vi "TPNT_ModifyDeviceTP.vi"(8 "error in (no error)":errorcluster, 9 "name":string, 10 "arguments":string, 11 "Object Refnum In":T1) -> (0 "error out":errorcluster, 3 "Data Refnum out":T1)   [LabVIEW 2016]
uses:
  TPNT_Refnum.ctl
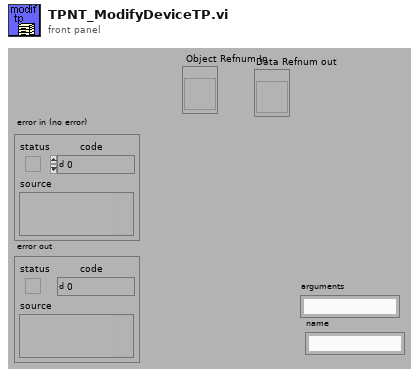
[diagram p1: front panel]
types:
  T1 = typedef "TPNT_Refnum.ctl" = refnum<vi>
  T2 = typedef "TPNT_TP.ctl" = cluster{"name":string, "type":string, "algor":string[], "update_rate":sgl, "Limits":T3, "Samples":T4, "next_update":u32, "Status":string, "monitor":bool, "error":bool, "Log":T5, "permissions":string, "ID":string}
  T3 = typedef "TPNT_Limits.ctl" = cluster{"Alarm Type":string, "Lower ":dbl, "Upper":dbl, "Nominal":dbl, "outrange":bool, "Check":bool, "latch":bool, "level":string}
  T4 = typedef "TPNT_Samples.ctl" = cluster{"samples":i32, "counter":i32, "Values":dbl[], "Current Value":string, "filter":string, "precision":u8}
  T5 = typedef "TPNT_Log.ctl" = cluster{"log":bool, "file":path, "type":string, "format":string, "updaterate":dbl, "nex_update":u32, "mode":string}
  T6 = typedef "TPNT_DeviceTPs.ctl" = cluster{"device":string, "devupdate":dbl, "next_update":u32, "devinterface":string, "TPs":T2[], "Alarms":bool, "monitor":bool, "log sep":string}
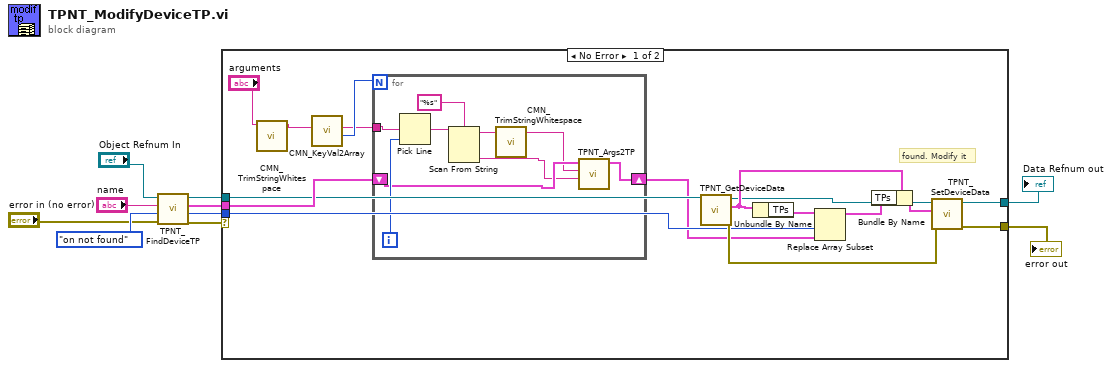
[diagram p0: block diagram]
diagram:
  n1 = call "TPNT_FindDeviceTP.vi"("error in (no error)"="error in (no error)", "error"=enum16{"none", "on found", "on not found"}."on not found", "TP name"="name", "Object Refnum In"="Object Refnum In") -> ("error out"=w8:errorcluster, "index"=w5:i32, "TP"=w6:T2, "Data Refnum out"=w3:T1)  [unwired: 4 out]
  n2 = case shown="No Error" w8 {
    selector: w8 -> [_ w37]
    tunnel: w6 -> [w22 _]
    tunnel: w5 -> [w14 _]
    tunnel: w3 -> [w15 w36]
    tunnel: [w12 w36] -> w2
    tunnel: [w11 w37] -> w1
    frame No Error {
      # "found. Modify it"
      n3 = call "CMN_TrimStringWhitespace.vi"("string"="arguments") -> ("trimmed string"=w23:string)  [unwired: 1 in, 8 out]
      n4 = call "CMN_KeyVal2Array.vi"("command in"=w23) -> ("number of commands"=w26:i32, "commands out"=w25:string)  [unwired: 2 in, 6 out]
      n5 = for {
        N: w26 -> [_]
        tunnel: w25 -> [w35]
        shift-right: [w29] -> w13
        shift-left: w22 -> [w30]
        i -> [w34]
        n6 = Pick Line(multi-line string=w35, line index=w34) -> (output string=w33:string)  [unwired: 1 out]
        n7 = Scan From String(format string="%s", input string=w33) -> (remaining string=w31:string, output 1=w27:string)  [unwired: 2 in, 3 out]
        n8 = call "CMN_TrimStringWhitespace.vi"("string"=w31) -> ("trimmed string"=w28:string)  [unwired: 1 in, 8 out]
        n9 = call "TPNT_Args2TP.vi"("key"=w27, "value"=w28, "TP_IN"=w30) -> ("TP_OUT"=w29:T2)  [unwired: 8 out]
      }
      n10 = call "TPNT_GetDeviceData.vi"("Object Refnum In"=w15) -> ("error out"=w16:errorcluster, "Object Data Out"=w19:T6, "Data Refnum out"=w18:T1)  [unwired: 1 in, 7 out]
      n11 = Unbundle By Name(w19) -> ("TPs"=w21:T2[])
      n12 = Replace Array Subset(array=w21, new element=w13, index=w14) -> (w20:T2[])
      n13 = Bundle By Name(cluster=w19, "TPs"=w20) -> (w17:T6)
      n14 = call "TPNT_SetDeviceData.vi"("error in (no error)"=w16, "Object Data In"=w17, "Object Refnum In"=w18) -> ("error out"=w11:errorcluster, "Data Refnum out"=w12:T1)  [unwired: 7 out]
    }
    frame Error {
    }
  }
  "error out" <- w1
  "Data Refnum out" <- w2
